vi "Test GUI.vi"() -> ()   [LabVIEW 2021, in "JSONTextViewer.lvlib"]
uses:
  JSONTextViewer.lvlib
  JSONTextViewer/JSONTextViewer.lvclass
panel:
  in  "stop":bool
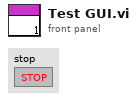
[diagram p1: front panel]
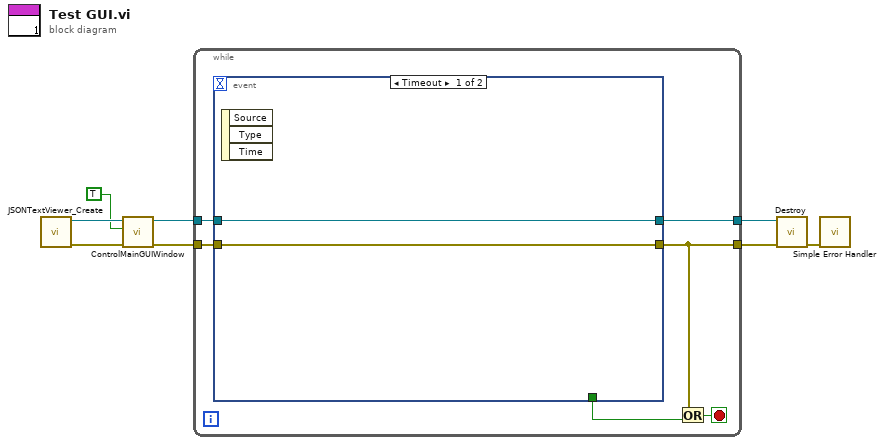
[diagram p0: block diagram]
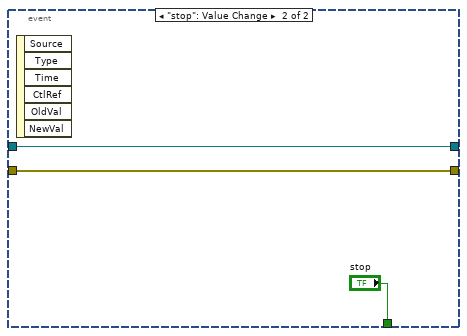
[diagram p2: hidden frame]
diagram:
  n1 = call "JSONTextViewer_Create.vi"() -> ("Error Out"=w7:errorcluster, "reference out"=w8:refnum<class "JSONTextViewer.lvclass">)  [unwired: 10 in]
  n2 = call "ControlMainGUIWindow.vi"("Error In"=w7, "ShowProcessWindow"=TRUE, "reference in"=w8) -> ("Error Out"=w5:errorcluster, "reference out"=w4:refnum<class "JSONTextViewer.lvclass">)  [unwired: 6 in, 1 out]
  n3 = while {
    tunnel: w5 -> [w14]
    tunnel: w4 -> [w13]
    tunnel: [w11] -> w3
    tunnel: [w9] -> w2
    stop <- w10 stop-if-true
    n4 = event shown="[0] Timeout" {
      selector: _ -> [_ _]
      dyn-events: _ -> [_ _]
      timeout: _ -> [_ _]
      tunnel: w14 -> [w15 w17]
      tunnel: w13 -> [w16 w18]
      tunnel: [_ "stop"] -> w12
      tunnel: [w16 w18] -> w11
      tunnel: [w15 w17] -> w9
      event Timeout {
        n5 = event-data() -> ()  [unwired: 1 in, 3 out]
      }
      event "stop": Value Change {
        n6 = event-data() -> ()  [unwired: 1 in, 6 out]
      }
    }
    n7 = Or(x=w9, y=w12) -> (x .or. y?=w10:bool)
  }
  n8 = call-dynamic "Destroy.vi"("Error In"=w2, "reference in"=w3) -> ("Error Out"=w1:errorcluster)  [unwired: 8 in, 1 out]
  n9 = call <vilib>:"Simple Error Handler.vi"("error in (no error)"=w1) -> ()  [unwired: 4 in, 5 out]
